vi "Ev Menu.vi"(8 "error in (no error)":errorcluster, 10 "ItemTag":string, 11 "LF2R IDE in":refnum<class "Main Panel.lvclass">) -> (0 "error out":errorcluster, 3 "LF2R IDE out":refnum<class "Main Panel.lvclass">)   [LabVIEW 2018, in "Main Panel.lvlib" / "Main Panel.lvclass"]
uses:
  Main Panel.lvclass
  Menu item.ctl
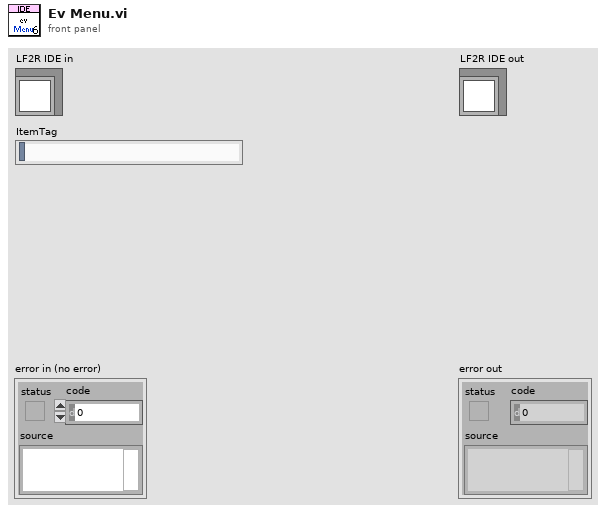
[diagram p1: front panel]
types:
  T1 = typedef "Main Panel.lvlib/Main Panel.lvclass/Menu item.ctl" = enum16{"Invalid Item", "File", "Open File", "Save File", "Exit", "Settings", "Preferences", "Help", "Show Context Help", "Tool", "Pic Json Generator"}
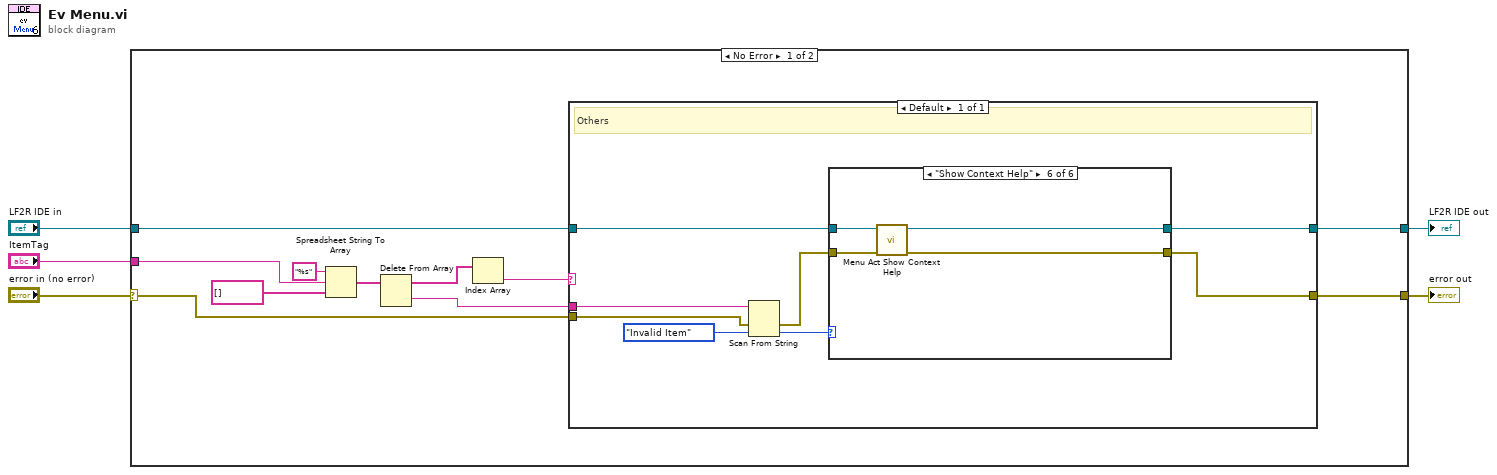
[diagram p0: block diagram]
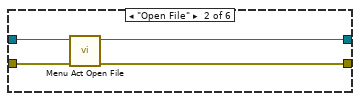
[diagram p3: hidden frame]
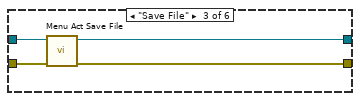
[diagram p4: hidden frame]
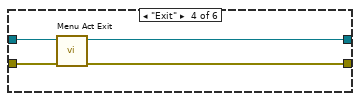
[diagram p5: hidden frame]
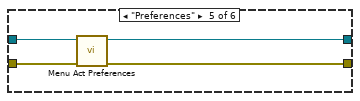
[diagram p6: hidden frame]
diagram:
  n1 = case shown="No Error" "error in (no error)" {
    selector: "error in (no error)" -> [w13 w48]
    tunnel: [w14 w48] -> w4
    tunnel: [w15 w47] -> w2
    tunnel: "LF2R IDE in" -> [w16 w47]
    tunnel: "ItemTag" -> [w12 _]
    frame No Error {
      n2 = Spreadsheet String To Array(format string="%s", spreadsheet string=w12, array type (2D Dbl)=string[] []) -> (array=w9:string[])  [unwired: 1 in]
      n3 = Delete From Array(array=w9) -> (deleted portion=w8:string, array with subset deleted=w7:string[])  [unwired: 2 in]
      n4 = Index Array(array=w7) -> (element=w6:string)  [unwired: 1 in]
      n5 = case shown="Default" w6 {
        tunnel: w16 -> [w22]
        tunnel: [w20] -> w15
        tunnel: [w19] -> w14
        tunnel: w13 -> [w18]
        tunnel: w8 -> [w17]
        frame Default {
          # "Others"
          n6 = Scan From String(input string=w17, error in=w18, default 1=Menu_item."Invalid Item" ("Menu item")) -> (error out=w21:errorcluster, output 1=w23:T1)  [unwired: 2 in, 2 out]
          n7 = case shown="\"Show Context Help\"" w23 {
            tunnel: w22 -> [w26 w30 w34 w38 w42 w46]
            tunnel: w21 -> [w25 w29 w33 w37 w41 w45]
            tunnel: [w26 w28 w32 w36 w39 w43] -> w20
            tunnel: [w25 w27 w31 w35 w40 w44] -> w19
            frame Default {
            }
            frame "Open File" {
              n8 = call "Menu Act Open File.vi"("error in (no error)"=w29, "LF2R IDE in"=w30) -> ("error out"=w27:errorcluster, "LF2R IDE out"=w28:refnum<class "Main Panel.lvclass">)  [unwired: 8 in]
            }
            frame "Save File" {
              n9 = call "Menu Act Save File.vi"("error in (no error)"=w33, "LF2R IDE in"=w34) -> ("error out"=w31:errorcluster, "LF2R IDE out"=w32:refnum<class "Main Panel.lvclass">)  [unwired: 8 in]
            }
            frame "Exit" {
              n10 = call "Menu Act Exit.vi"("error in (no error)"=w37, "LF2R IDE in"=w38) -> ("error out"=w35:errorcluster, "LF2R IDE out"=w36:refnum<class "Main Panel.lvclass">)  [unwired: 8 in]
            }
            frame "Preferences" {
              n11 = call "Menu Act Preferences.vi"("error in (no error)"=w41, "LF2R IDE in"=w42) -> ("error out"=w40:errorcluster, "LF2R IDE out"=w39:refnum<class "Main Panel.lvclass">)  [unwired: 8 in]
            }
            frame "Show Context Help" {
              n12 = call "Menu Act Show Context Help.vi"("error in (no error)"=w45, "LF2R IDE in"=w46) -> ("error out"=w44:errorcluster, "LF2R IDE out"=w43:refnum<class "Main Panel.lvclass">)  [unwired: 8 in]
            }
          }
        }
      }
    }
    frame Error {
    }
  }
  "error out" <- w4
  "LF2R IDE out" <- w2
